vi "PH_Calorimeter_USB.Set GUI elements.vi"(0 "i ref in":refnum<vi>, 5 "error in (no error)":errorcluster) -> (14 "i ref out":refnum<vi>, 19 "error out":errorcluster)   [LabVIEW 2014, in "PH_Calorimeter_USB.lvlib"]
doc: "This VI gets information from the data base and input, sets the attributes and the related GUI elements."
uses:
  PH_Calorimeter_USB.lvlib
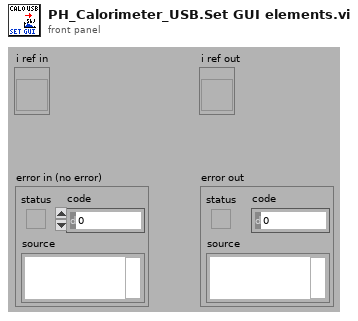
[diagram p1: front panel]
types:
  T1 = typedef "PH_Calorimeter_USB.lvlib/PH_Calorimeter_USB.i attribute.ctl" = cluster{"GUI Refs":cluster{"Delete":refnum<vi>, "Start":refnum<vi>, "Energy":refnum<vi>, "Calorimeter":refnum<vi>, "Trigger":refnum<vi>, "Calo Calibration":refnum<vi>, "Time Base":refnum<vi>, "Device":refnum<vi>, "Graph Raw Data":refnum<vi>, "Graph Result":refnum<vi>}, "DAQ Instance":string, "Data":dbl[][], "Controller Instance":string, "Energy [J]":dbl, "Calorimeter":T2, "Trigger":T3, "Time Base":T4, "Calo Calibration":T5, "Serial Number":string}
  T2 = typedef "PH_Calorimeter_USB.lvlib/PH_Calorimeter_USB.Calorimeter Settings.ctl" = cluster{"Channel":tag, "Min Value [V]":dbl, "Max Value  [V]":dbl}
  T3 = typedef "PH_Calorimeter_USB.lvlib/PH_Calorimeter_USB.Trigger Settings.ctl" = cluster{"Channel":tag, "Min Value [V]":dbl, "Max Value  [V]":dbl, "Level [V]":dbl, "Wait Time [s]":dbl, "Length [Samples]":i32}
  T4 = typedef "PH_Calorimeter_USB.lvlib/PH_Calorimeter_USB.Time Base Settings.ctl" = cluster{"Samples per Channel":i32, "Rate [Hz]":i32}
  T5 = typedef "PH_Calorimeter_USB.lvlib/PH_Calorimeter_USB.Calorimeter Calibration Settings.ctl" = cluster{"T 1/e [s]":dbl, "Sensitivity  [Vs/J]":dbl}
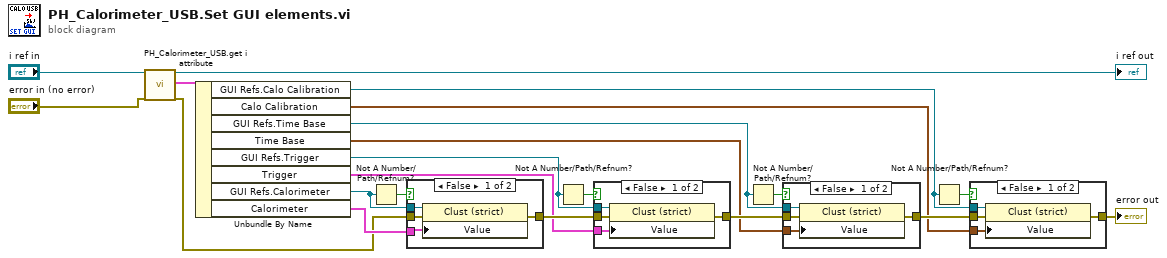
[diagram p0: block diagram]
diagram:
  n1 = call "PH_Calorimeter_USB.get i attribute.vi"("i ref in"="i ref in", "error in (no error)"="error in (no error)") -> ("i ref out"=→"i ref out":refnum<vi>, "i attribute"=w9:T1, "error out"=w1:errorcluster)  [unwired: 15 in]
  n2 = Unbundle By Name(w9) -> ("GUI Refs.Calo Calibration"=w11:refnum<vi>, "Calo Calibration"=w10:T5, "GUI Refs.Time Base"=w3:refnum<vi>, "Time Base"=w2:T4, "GUI Refs.Trigger"=w5:refnum<vi>, "Trigger"=w4:T3, "GUI Refs.Calorimeter"=w7:refnum<vi>, "Calorimeter"=w6:T2)
  n3 = Not A Number/Path/Refnum?(number/path/refnum=w7) -> (NaN/Path/Refnum?=w18:bool)
  n4 = case shown="False" w18 {
    tunnel: w1 -> [w25 w26]
    tunnel: [w24 w26] -> w12
    tunnel: w7 -> [w23 _]
    tunnel: w6 -> [w22 _]
    frame False {
      n5 = property class="Clust (strict)"(reference=w23, error in=w25, "Value"=w22) -> (error out=w24:errorcluster)  [unwired: 1 out]
    }
    frame True {
    }
  }
  n6 = Not A Number/Path/Refnum?(number/path/refnum=w5) -> (NaN/Path/Refnum?=w17:bool)
  n7 = case shown="False" w17 {
    tunnel: w12 -> [w30 w31]
    tunnel: [w29 w31] -> w14
    tunnel: w5 -> [w28 _]
    tunnel: w4 -> [w27 _]
    frame False {
      n8 = property class="Clust (strict)"(reference=w28, error in=w30, "Value"=w27) -> (error out=w29:errorcluster)  [unwired: 1 out]
    }
    frame True {
    }
  }
  n9 = Not A Number/Path/Refnum?(number/path/refnum=w3) -> (NaN/Path/Refnum?=w16:bool)
  n10 = case shown="False" w16 {
    tunnel: w14 -> [w35 w36]
    tunnel: [w34 w36] -> w13
    tunnel: w3 -> [w33 _]
    tunnel: w2 -> [w32 _]
    frame False {
      n11 = property class="Clust (strict)"(reference=w33, error in=w35, "Value"=w32) -> (error out=w34:errorcluster)  [unwired: 1 out]
    }
    frame True {
    }
  }
  n12 = Not A Number/Path/Refnum?(number/path/refnum=w11) -> (NaN/Path/Refnum?=w15:bool)
  n13 = case shown="False" w15 {
    tunnel: w13 -> [w40 w41]
    tunnel: [w39 w41] -> w20
    tunnel: w11 -> [w38 _]
    tunnel: w10 -> [w37 _]
    frame False {
      n14 = property class="Clust (strict)"(reference=w38, error in=w40, "Value"=w37) -> (error out=w39:errorcluster)  [unwired: 1 out]
    }
    frame True {
    }
  }
  "error out" <- w20
